vi "zadanie 3_ciag_Fibonacciego.vi"() -> ()   [LabVIEW 2018]
panel:
  out "kolejne liczby ciagu":dbl[](array[numeric])
  out "N-ty element ciagu Fibonacciego":dbl
  in  "podaj ktory element ma byc wyœwietlony":i32
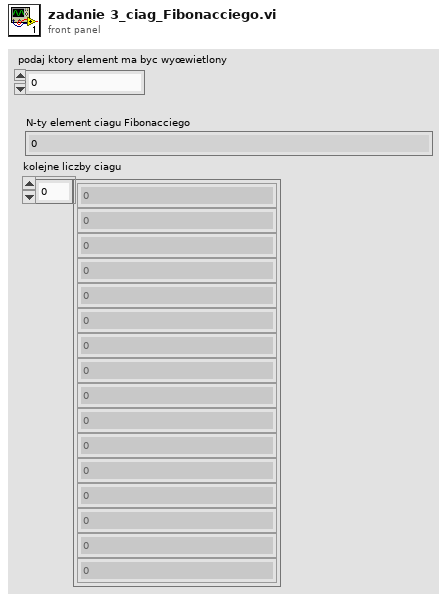
[diagram p1: front panel]
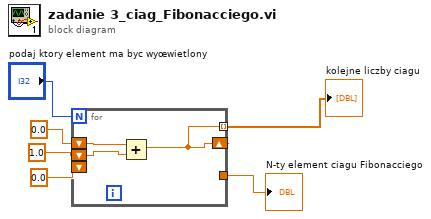
[diagram p0: block diagram]
diagram:
  n1 = for {
    N: "podaj ktory element ma byc wyœwietlony" -> [_]
    shift-right: [w7] -> _
    shift-left: 1.0 -> [w8]
    shift-left: 0.0 -> [_]
    tunnel: [w7] -> w5
    shift-left: 0.0 -> [w9]
    tunnel: [w7] -> w1 mode=indexing
    n2 = Add(x=w9, y=w8) -> (x+y=w7:dbl)
  }
  "N-ty element ciagu Fibonacciego" <- w5
  "kolejne liczby ciagu" <- w1
